vi "PositionBased1DProfile.vi"(9 "MaxAccel":dbl, 10 "MaxVel":dbl, 11 "Distance":dbl) -> (3 "Profile":cluster{"Distances":dbl[], "Vels":dbl[]})   [LabVIEW 2017]
panel:
  out "XY Graph":cluster{dbl[], dbl[]}(graph)
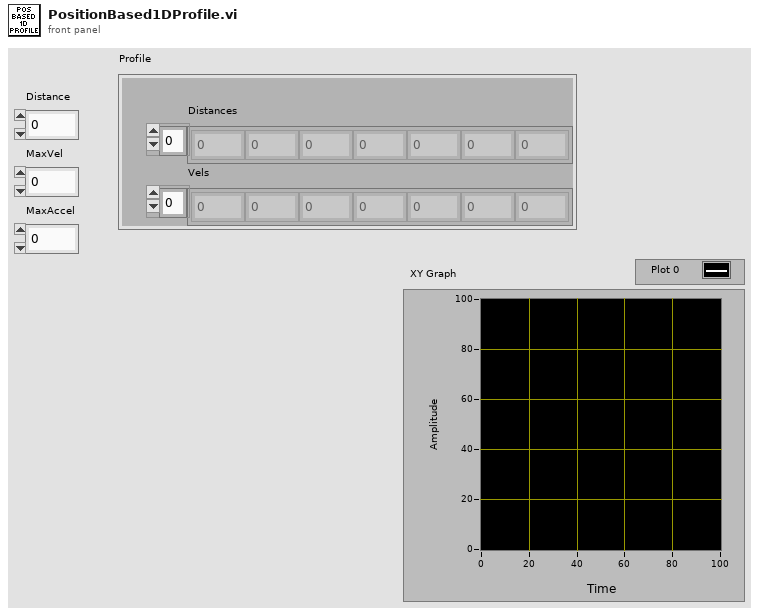
[diagram p1: front panel]
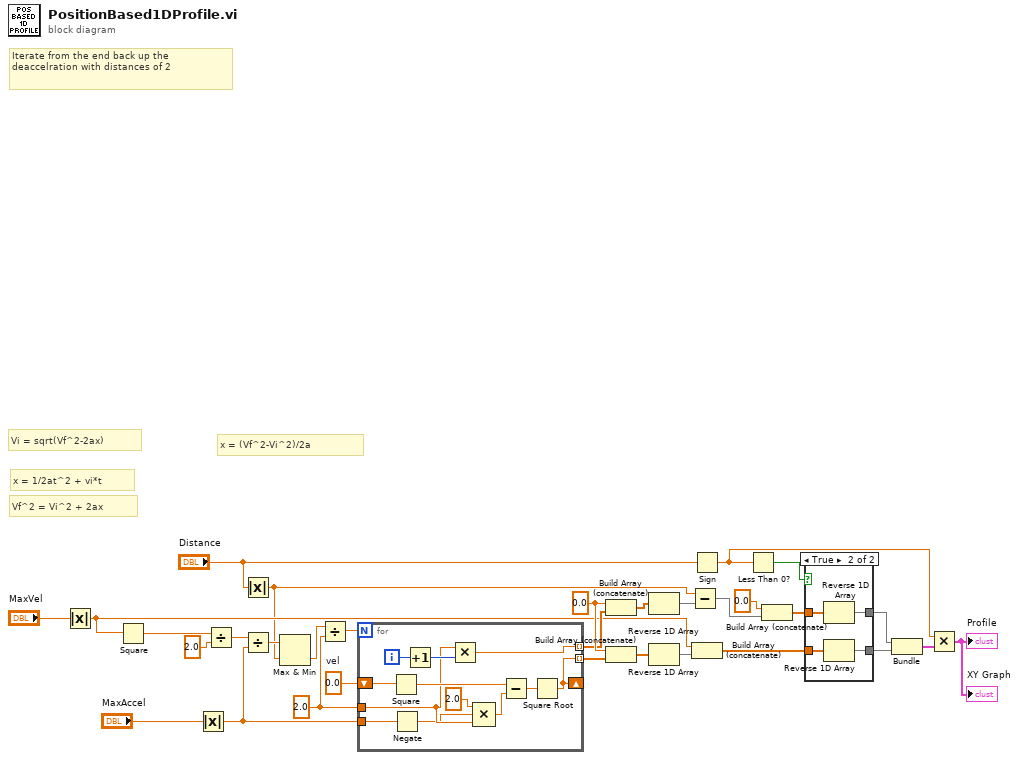
[diagram p0: block diagram]
diagram:
  w23 = 0.0 ("y")
  w27 = 0.0  # vel
  w28 = 2.0 ("y")
  # "Vi = sqrt(Vf^2-2ax)"
  # "Iterate from the end back up the\ndeaccelration with distances of 2"
  # "x = (Vf^2-Vi^2)/2a"
  # "Vf^2 = Vi^2 + 2ax"
  # "x = 1/2at^2 + vi*t"
  n1 = Absolute Value(x="MaxVel") -> (abs(x)=w13:dbl)
  n2 = Square(x=w13) -> (x^2=w29:dbl)
  n3 = Absolute Value(x="MaxAccel") -> (abs(x)=w11:dbl)
  n4 = Divide(x=w29, y=2.0) -> (x/y=w30:dbl)
  n5 = Absolute Value(x="Distance") -> (abs(x)=w10:dbl)
  n6 = Divide(x=w30, y=w11) -> (x/y=w25:dbl)
  n7 = Max & Min(x=w25, y=w10) -> (min(x,y)=w16:dbl)  [unwired: 1 out]
  n8 = Divide(x=w16, y=w28) -> (x/y=w24:dbl)
  n9 = for {
    N: w24 -> [_]
    tunnel: w28 -> [w38]
    shift-right: [w35] -> _
    shift-left: w27 -> [w41]
    tunnel: w11 -> [w34]
    tunnel: [w35] -> w22 mode=indexing
    tunnel: [w32] -> w21 mode=indexing
    i -> [w43]
    n10 = Square(x=w41) -> (x^2=w40:dbl)
    n11 = Negate(x=w34) -> (-x=w33:dbl)
    n12 = Increment(x=w43) -> (x+1=w42:i32)
    n13 = Multiply(x=w38, y=w42) -> (x*y=w32:dbl)
    n14 = Compound Arithmetic op=MULTIPLY(2.0 ("value"), w33, w38) -> (w37:dbl)
    n15 = Subtract(x=w40, y=w37) -> (x-y=w36:dbl)
    n16 = Square Root(x=w36) -> (sqrt(x)=w35:dbl)
  }
  n17 = Build Array (concatenate)(w23, w21) -> (w20:dbl[])
  n18 = Build Array (concatenate)(w23, w22) -> (w26:dbl[])
  n19 = Reverse 1D Array(array=w20) -> (reversed array=w17:dbl[])
  n20 = Reverse 1D Array(array=w26) -> (reversed array=w18:dbl[])
  n21 = Subtract(x=w10, y=w17) -> (x-y=w15:dbl[])
  n22 = Sign(1:"Distance") -> (0:w6:dbl)
  n23 = Build Array (concatenate)(w13, w18) -> (w3:dbl[])
  n24 = Less Than 0?(x=w6) -> (x < 0?=w1:bool)
  n25 = Build Array (concatenate)(0.0 ("y"), w15) -> (w4:dbl[])
  n26 = case shown="True" w1 {
    tunnel: [w45 w48] -> w5
    tunnel: w4 -> [w45 w49]
    tunnel: w3 -> [w44 w47]
    tunnel: [w44 w46] -> w2
    frame False {
    }
    frame True {
      n27 = Reverse 1D Array(array=w49) -> (reversed array=w48:dbl[])
      n28 = Reverse 1D Array(array=w47) -> (reversed array=w46:dbl[])
    }
  }
  n29 = Bundle(w5, w2) -> (w8:cluster{dbl[], dbl[]})  [unwired: 1 in]
  n30 = Multiply(x=w6, y=w8) -> (x*y=→"Profile" →"XY Graph":cluster{dbl[], dbl[]})
